vi "Initialize.vi"(8 "Error In":errorcluster, 11 "Display Manager In":refnum<class "Display Manager.lvclass">) -> (0 "Error Out":errorcluster, 3 "Display Manager Out":refnum<class "Display Manager.lvclass">)   [LabVIEW 2019, in "Display Manager.lvclass"]
uses:
  Display Manager.lvclass
  Process/Process.lvclass
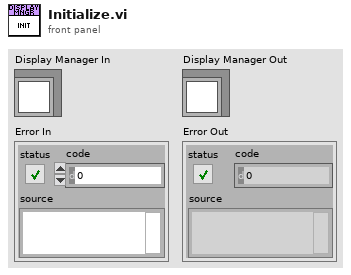
[diagram p1: front panel]
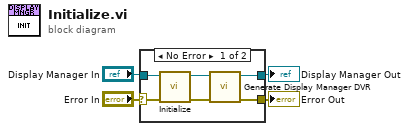
[diagram p0: block diagram]
diagram:
  n1 = case shown="No Error" "Error In" {
    selector: "Error In" -> [w10 w11]
    tunnel: [w6 w11] -> w4
    tunnel: [w5 w12] -> w3
    tunnel: "Display Manager In" -> [w9 w12]
    frame No Error {
      n2 = call-parent "Initialize.vi"("Error In"=w10, "Process In"=w9) -> ("Error Out"=w7:errorcluster, "Process Out"=w8:refnum<class "Display Manager.lvclass">)  [unwired: 8 in]
      n3 = call "Generate Display Manager DVR.vi"("Error In"=w7, "Display Manager In"=w8) -> ("Error Out"=w6:errorcluster, "Display Manager Out"=w5:refnum<class "Display Manager.lvclass">)  [unwired: 8 in]
    }
    frame Error {
    }
  }
  "Display Manager Out" <- w3
  "Error Out" <- w4
